vi "Stop Core.vi"(10 "final error code":i32, 11 "IED Status Logger in":refnum<class "IED Status Logger.lvclass">) -> (3 "IED Status Logger out":refnum<class "IED Status Logger.lvclass">)   [LabVIEW 2018, in "IED Status Logger Actor.lvlib" / "IED Status Logger.lvclass"]
doc: "(<B>Filename</B>: Actor Framework.lvlib:Actor.lvclass:Stop Core.vi)\n\nDefines what the actor does before it stops. Use the <B>final error code</B> input to determine whether the actor shut down in response to an error.\n\nBy default, this method does nothing. A descendant class may override it to define behavior, such as shutting down any processes the actor initiated in its override of the Actor Core method."
uses:
  IED Status Logger.lvclass
  IED Status Logger.lvclass/IED Status Logger.ctl
  <vilib>/ActorFramework/Actor/Actor.lvclass
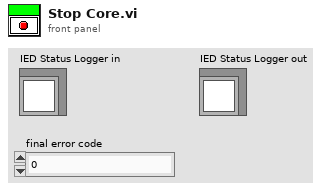
[diagram p1: front panel]
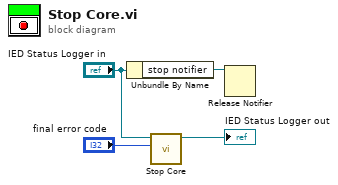
[diagram p0: block diagram]
diagram:
  n1 = Unbundle By Name("IED Status Logger in") -> ("stop notifier"=w1:refnum<notifier>)
  n2 = call-parent "Stop Core.vi"("final error code"="final error code", "Actor in"="IED Status Logger in") -> ("Actor out"=→"IED Status Logger out":refnum<class "IED Status Logger.lvclass">)  [unwired: 9 in]
  n3 = Release Notifier(notifier=w1) -> ()  [unwired: 2 in, 3 out]
